vi "IIR Filter with I.C..vi"   [LabVIEW 2017, in "NI_AALBase.lvlib"]
doc: "Filters the input sequence <B>X</B> using the direct form IIR filter specified by <B>Reverse Coefficients</B> and <B>Forward Coefficients</B>. You can use this VI to process blocks of continuous data. This VI is similar to the IIR Filter VI except that you specify the initial conditions for this VI. Wire data to the <B>X</B> input to determine the polymorphic instance to use or manually select the instance."
uses:
  NI_AALBase.lvlib
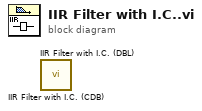
[diagram p0: block diagram]
diagram:
  n1 = call "IIR Filter with I.C. (CDB).vi"() -> ()  [unwired: 7 in, 4 out]
  n2 = call "IIR Filter with I.C. (DBL).vi"() -> ()  [unwired: 7 in, 4 out]
